vi "Object Tracking.vi"() -> ()   [LabVIEW 2014]
doc: "This example demonstrates the Traditional MeanShift algorithm to track an object in the image."
panel:
  in  "Stop":bool
  in  "Delay (s.)":dbl(slide) scale=0.0..2.0
  out "Image":T1(plugin-control)
  # "Overview: Demonstrate the Traditional MeanShift algorithm to track an object in the image.\nRequirements: LabVIEW Full Development System and Vision Development Module.\nInstructions: Run the VI."
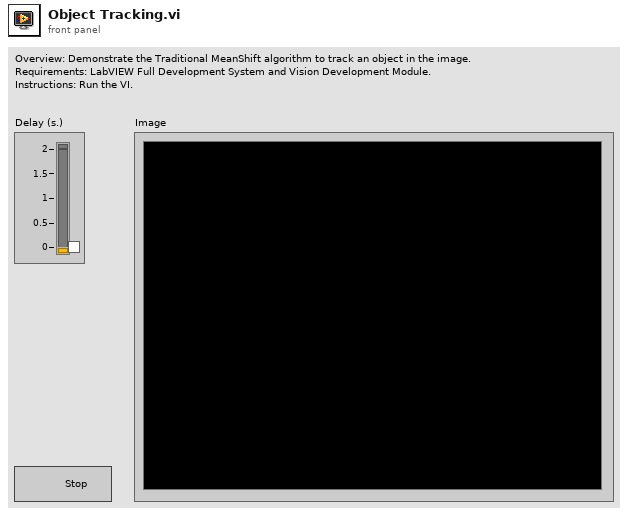
[diagram p1: front panel]
types:
  T1 = typedef "IMAQ Image.ctl" = refnum<image>
  T2 = cluster{"Number of Histogram Bins":i32, "Blending Parameter (%)":dbl, "Maximum Iterations":i32}
  T3 = typedef "Image Type" = u32
  T4 = typedef "IMAQ Object Tracking Session.ctl" = refnum<k20>
  T5 = typedef "IMAQ AVI2 Refnum.ctl" = refnum<k20>
  T6 = typedef "IMAQ Rectangle" = cluster{"Left":i32, "Top":i32, "Right":i32, "Bottom":i32, "Rotation":dbl}
  T7 = typedef "ROI Descriptor" = cluster{"Global Rectangle":i32[], "Contours":cluster{"ID":enum32{"External", "Internal"}, "Type":u32, "Coordinates":i32[]}[]}
  T8 = cluster{"Label":string, "Score":i32, "Angle":dbl, "Location":cluster{"X":dbl, "Y":dbl}, "Bounding Box":cluster{"X":dbl, "Y":dbl}[], "Object Found?":bool}[]
  T9 = cluster{"Label":string, "Score":i32, "Angle":dbl, "Location":cluster{"X":dbl, "Y":dbl}, "Bounding Box":cluster{"X":dbl, "Y":dbl}[], "Object Found?":bool}
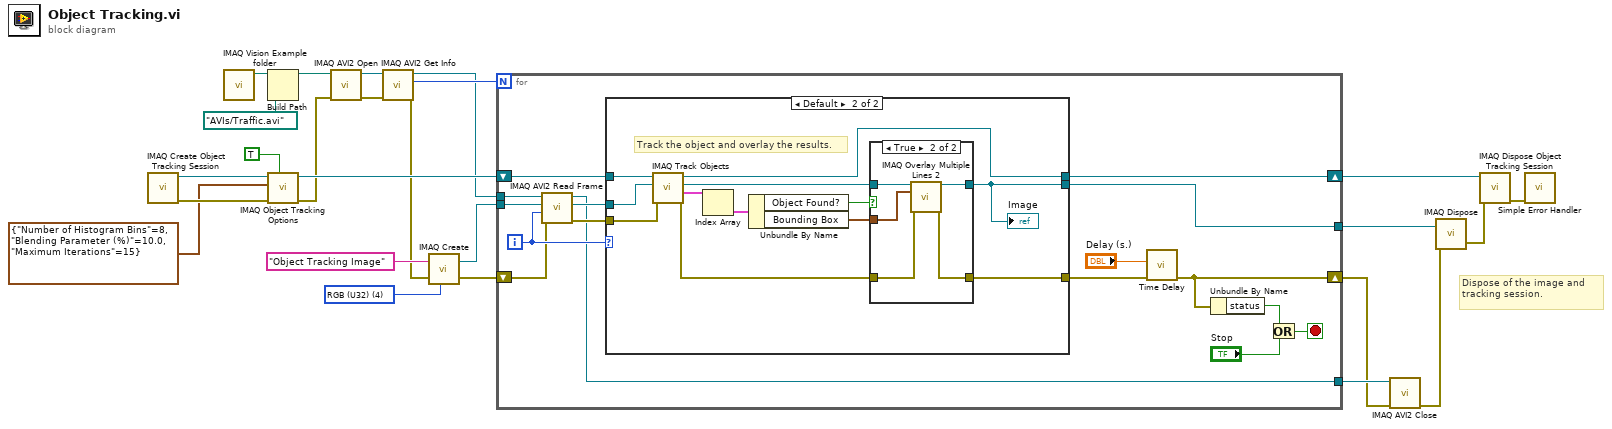
[diagram p0: block diagram]
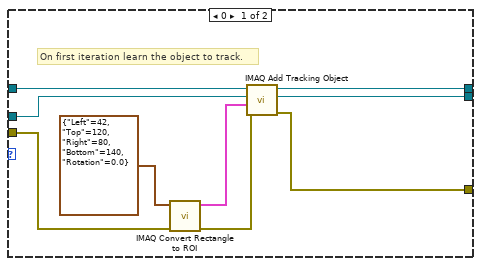
[diagram p2: hidden frame]
diagram:
  w8 = T3 4 items=["Grayscale (U8)", "Grayscale (I16)", "Grayscale (SGL)", "Complex (CSG)", "RGB (U32)", "HSL (U32)", "RGB (U64)", "Grayscale (U16)"] ("Image Type")
  # "Dispose of the image and tracking session."
  n1 = call "IMAQ Create Object Tracking Session"() -> ("error out"=w16:errorcluster, "Object Tracking Session"=w19:T4)  [unwired: 1 in, 9 out]
  n2 = call "IMAQ Vision Example folder.vi"() -> ("Example Image Path"=w21:path)  [unwired: 11 in]
  n3 = Build Path(base path=w21, name or relative path=path "AVIs/Traffic.avi" ("appended path")) -> (appended path=w15:path)
  n4 = call-poly "IMAQ Object Tracking Options"("Get/Set (Get)"=TRUE, "error in (no error)"=w16, "Mean Shift Options in"=T2 {"Number of Histogram Bins"=8, "Blending Parameter (%)"=10.0, "Maximum Iterations"=15}, "Object Tracking Session In"=w19) -> ("error out"=w14:errorcluster, "Object Tracking Session Out"=w18:T4)  [unwired: 5 in, 1 out]
  n5 = call "IMAQ AVI2 Open"("error in (no error)"=w14, "AVI File Path"=w15) -> ("error out"=w12:errorcluster, "AVI Refnum"=w13:T5)  [unwired: 8 in]
  n6 = call "IMAQ AVI2 Get Info"("error in (no error)"=w12, "AVI Refnum"=w13) -> ("error out"=w9:errorcluster, "Number of Frames"=w11:u32, "AVI Refnum (duplicate)"=w7:T5)  [unwired: 5 in, 2 out]
  n7 = call "IMAQ Create"("Image Name"="Object Tracking Image", "Image Type"=w8, "error in (no error)"=w9) -> ("New Image"=w6:T1, "error out"=w5:errorcluster)  [unwired: 2 in]
  n8 = for {
    N: w11 -> [_]
    tunnel: [w40] -> w25
    shift-right: [w38] -> w24
    shift-left: w18 -> [w39]
    tunnel: w7 -> [w35]
    tunnel: w6 -> [w34]
    shift-right: [w27] -> w3
    shift-left: w5 -> [w28]
    tunnel: [w26] -> w4
    i -> [w31]
    stop <- w29 stop-if-true
    n9 = call "IMAQ AVI2 Read Frame"("error in (no error)"=w28, "Frame Number"=w31, "Image"=w34, "AVI Refnum"=w35) -> ("error out"=w32:errorcluster, "Image Out"=w33:T1, "AVI Refnum (duplicate)"=w26:T5)  [unwired: 5 in]
    n10 = case shown="Default" w31 {
      tunnel: [w47 w62] -> w38
      tunnel: [w49 w59] -> w40
      tunnel: [w48 w55] -> w36
      tunnel: w39 -> [w50 w57]
      tunnel: w33 -> [w46 w53]
      tunnel: w32 -> [w45 w52]
      frame 0 {
        # "On first iteration learn the object to track."
        n11 = call "IMAQ Convert Rectangle to ROI"("error in (no error)"=w45, "Rectangle"=T6 {"Left"=42, "Top"=120, "Right"=80, "Bottom"=140, "Rotation"=0.0}) -> ("error out"=w44:errorcluster, "ROI Descriptor"=w43:T7)  [unwired: 7 in]
        n12 = call "IMAQ Add Tracking Object"("error in (no error)"=w44, "ROI Descriptor"=w43, "Image"=w46, "Object Tracking Session In"=w50) -> ("error out"=w48:errorcluster, "Image (duplicate)"=w49:T1, "Object Tracking Session Out"=w47:T4)  [unwired: 1 in, 4 out]
      }
      frame Default {
        # "Track the object and overlay the results."
        n13 = call "IMAQ Track Objects"("error in (no error)"=w52, "Image"=w53, "Object Tracking Session In"=w57) -> ("error out"=w56:errorcluster, "Objects (pixel)"=w61:T8, "Image (duplicate)"=w60:T1, "Object Tracking Session Out"=w62:T4)  [unwired: 1 in, 4 out]
        n14 = Index Array(array=w61) -> (element=w54:T9)  [unwired: 1 in]
        n15 = Unbundle By Name(w54) -> ("Object Found?"=w51:bool, "Bounding Box"=w58:cluster{"X":dbl, "Y":dbl}[])
        n16 = case shown="True" w51 {
          tunnel: w60 -> [w63 w69]
          tunnel: [w63 w68] -> w59
          tunnel: w58 -> [_ w67]
          tunnel: w56 -> [w64 w66]
          tunnel: [w64 w65] -> w55
          frame False {
          }
          frame True {
            n17 = call "IMAQ Overlay Multiple Lines 2"("Image"=w69, "Line End Points"=w67, "error in (no error)"=w66) -> ("Image Out"=w68:T1, "error out"=w65:errorcluster)  [unwired: 5 in, 6 out]
          }
        }
        "Image" <- w59
      }
    }
    n18 = call "Time Delay"("error in (no error)"=w36, "Delay Time (s)"="Delay (s.)") -> ("error out"=w27:errorcluster)  [unwired: 9 in]
    n19 = Unbundle By Name(w27) -> ("status"=w41:bool)
    n20 = Or(x=w41, y="Stop") -> (x .or. y?=w29:bool)
  }
  n21 = call "IMAQ AVI2 Close"("error in (no error)"=w3, "AVI Refnum"=w4) -> ("error out"=w2:errorcluster)  [unwired: 9 in]
  n22 = call "IMAQ Dispose"("Image"=w25, "error in (no error)"=w2) -> ("error out"=w23:errorcluster)  [unwired: 1 in, 3 out]
  n23 = call "IMAQ Dispose Object Tracking Session"("error in (no error)"=w23, "Object Tracking Session"=w24) -> ("error out"=w22:errorcluster)  [unwired: 9 out]
  n24 = call <vilib>:"Simple Error Handler.vi"("error in (no error)"=w22) -> ()  [unwired: 1 in, 8 out]
